vi "PowerControl.vi"(8 "error in (no error)":errorcluster, 9 "Numeric":dbl, 10 "PowerType":enum16{"Itech", "Keysight"}(ring), 11 "PowerPort":string) -> (0 "error out":errorcluster, 2 "Fb":string)   [LabVIEW 2018]
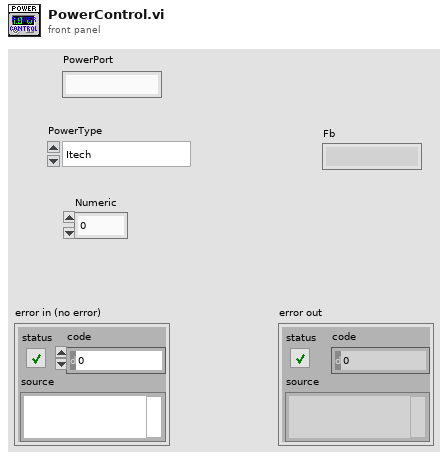
[diagram p1: front panel]
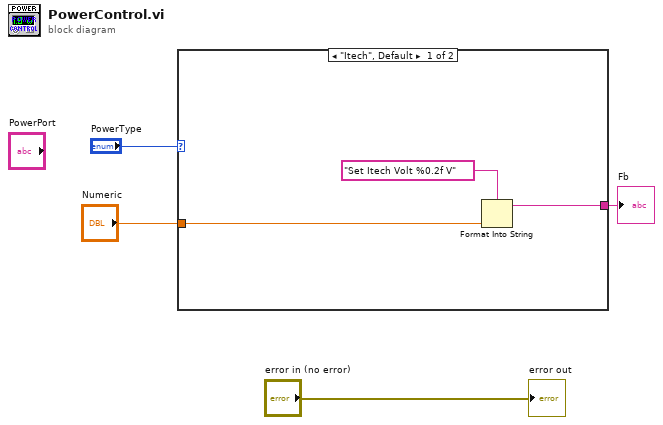
[diagram p0: block diagram]
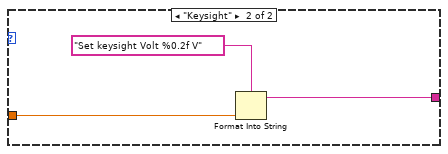
[diagram p2: hidden frame]
diagram:
  n1 = case shown="\"Itech\", Default" "PowerType" {
    tunnel: "Numeric" -> [w6 w10]
    tunnel: [w5 w8] -> w2
    frame "Itech", Default {
      n2 = Format Into String(format string="Set Itech Volt %0.2f V", w6) -> (resulting string=w5:string)  [unwired: 2 in, 1 out]
    }
    frame "Keysight" {
      n3 = Format Into String(format string="Set keysight Volt %0.2f V", w10) -> (resulting string=w8:string)  [unwired: 2 in, 1 out]
    }
  }
  "Fb" <- w2
  "error out" <- "error in (no error)"
